vi "Get Path Regex.vi"(8 "error in (no error)":errorcluster, 11 "Submit in":refnum<class "Submit.lvclass">) -> (0 "error out":errorcluster, 2 "Path Regex":string, 3 "Submit out":refnum<class "Submit.lvclass">)   [LabVIEW 2020, in "Summer of LabVIEW.lvlib" / "Submit.lvclass"]
uses:
  Submit.lvclass
  Submit.lvclass/Submit.ctl
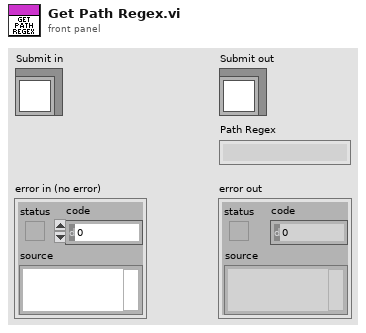
[diagram p1: front panel]
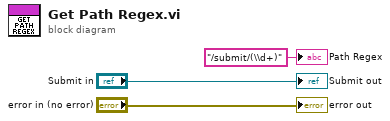
[diagram p0: block diagram]
diagram:
  "error out" <- "error in (no error)"
  "Submit out" <- "Submit in"
  "Path Regex" <- "/submit/(\\d+)" ("Path Regex")
